vi "Day 08 (Part One).vi"() -> ()   [LabVIEW 2021]
panel:
  out "result":i32
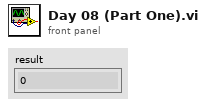
[diagram p1: front panel]
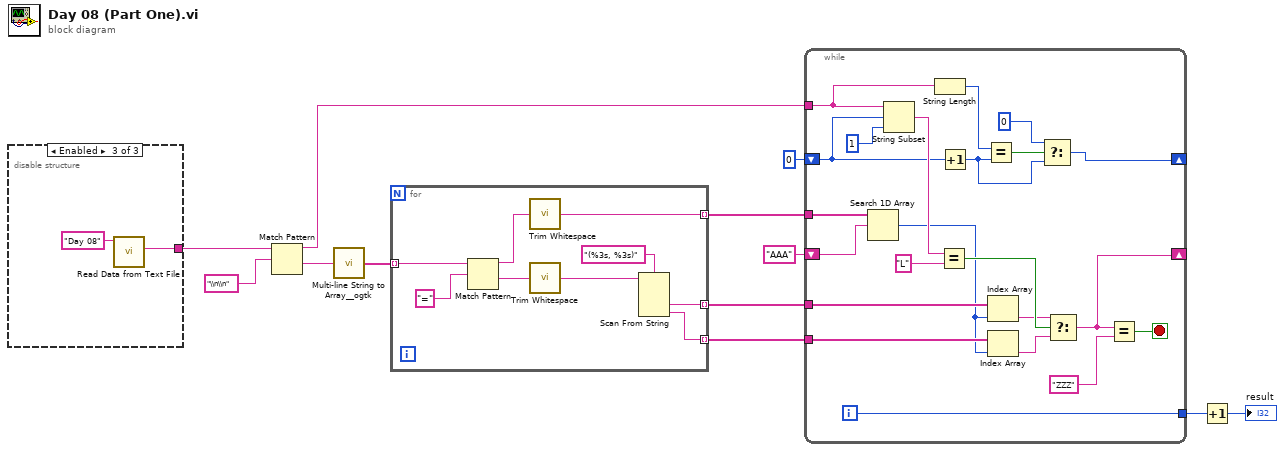
[diagram p0: block diagram]
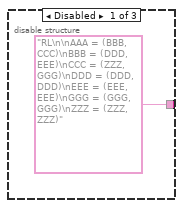
[diagram p2: hidden frame]
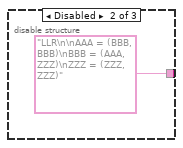
[diagram p3: hidden frame]
diagram:
  n1 = disable-structure shown="Enabled" {
    disable-tunnel: ["RL\n\nAAA = (BBB, CCC)\nBBB = (DDD, EEE)\nCCC = (ZZZ, GGG)\nDDD = (DDD, DDD)\nEEE = (EEE, EEE)\nGGG = (GGG, GGG)\nZZZ = (ZZZ, ZZZ)" "LLR\n\nAAA = (BBB, BBB)\nBBB = (AAA, ZZZ)\nZZZ = (ZZZ, ZZZ)" w16] -> w12
    frame Disabled {
    }
    frame Disabled {
    }
    frame Enabled {
      n2 = call "Read Data from Text File.vi"("Subfolder"="Day 08") -> ("data"=w16:string)  [unwired: 10 in]
    }
  }
  n3 = Match Pattern(string=w12, regular expression="\\n\\n") -> (before substring=w2:string, after substring=w10:string)  [unwired: 1 in, 2 out]
  n4 = call <userlib>:"Multi-line String to Array__ogtk.vi"("string"=w10) -> ("lines"=w9:string[])
  n5 = for {
    tunnel: w9 -> [w25] mode=indexing
    tunnel: [w19] -> w3 mode=indexing
    tunnel: [w18] -> w8 mode=indexing
    tunnel: [w17] -> w7 mode=indexing
    n6 = Match Pattern(string=w25, regular expression="=") -> (before substring=w23:string, after substring=w22:string)  [unwired: 1 in, 2 out]
    n7 = call <vilib>:"Trim Whitespace.vi"("string"=w23) -> ("trimmed string"=w19:string)  [unwired: 1 in]
    n8 = call <vilib>:"Trim Whitespace.vi"("string"=w22) -> ("trimmed string"=w20:string)  [unwired: 1 in]
    n9 = Scan From String(format string="(%3s, %3s)", input string=w20) -> (output 1=w18:string, output 2=w17:string)  [unwired: 4 in, 3 out]
  }
  n10 = while {
    tunnel: w8 -> [w40]
    tunnel: w7 -> [w39]
    shift-right: [w27] -> _
    shift-left: "AAA" -> [w44]
    tunnel: w3 -> [w45]
    shift-right: [w38] -> _
    shift-left: 0 ("t") -> [w29]
    tunnel: [w33] -> w5
    tunnel: w2 -> [w31]
    i -> [w33]
    stop <- w26 stop-if-true
    n11 = Search 1D Array(1D array=w45, element=w44) -> (index of element=w28:i32)  [unwired: 1 in]
    n12 = String Subset(string=w31, offset (0)=w29, length (rest)=1 ("length (rest)")) -> (substring=w37:string)
    n13 = String Length(string=w31) -> (length=w30:i32)
    n14 = Equal?(x=w37, y="L") -> (x = y?=w46:bool)
    n15 = Increment(x=w29) -> (x+1=w42:i32)
    n16 = Equal?(x=w30, y=w42) -> (x = y?=w43:bool)
    n17 = Index Array(array=w40, index=w28) -> (element=w35:string)
    n18 = Index Array(array=w39, index=w28) -> (element=w34:string)
    n19 = Select(t=0, s=w43, f=w42) -> (s? t:f=w38:i32)
    n20 = Select(t=w35, s=w46, f=w34) -> (s? t:f=w27:string)
    n21 = Equal?(x=w27, y="ZZZ") -> (x = y?=w26:bool)
  }
  n22 = Increment(x=w5) -> (x+1=→"result":i32)
